vi "Convert to Lockin Data.vi"(8 "error in (no error)":errorcluster, 10 "Raw data":i32[](array[numeric])=[67108864, 0, 0, 67108864, 0, 0, 67108864], 11 "RP Transceiver in":refnum<class "RP Transceiver.lvclass">) -> (0 "error out":errorcluster, 1 "Volatge X out":dbl[](array[numeric]), 2 "Frequency out":dbl[](array[numeric]), 3 "RP Transceiver out":refnum<class "RP Transceiver.lvclass">, 4 "Starting edges":i32[](array[numeric]), 5 "Ending edges":i32[](array[numeric]), 6 "Volatge Y out":dbl[](array[numeric]))   [LabVIEW 2016, in "RP Transceiver.lvclass"]
uses:
  RP Transceiver.lvclass
  RP Transceiver.lvclass/RP Transceiver.ctl
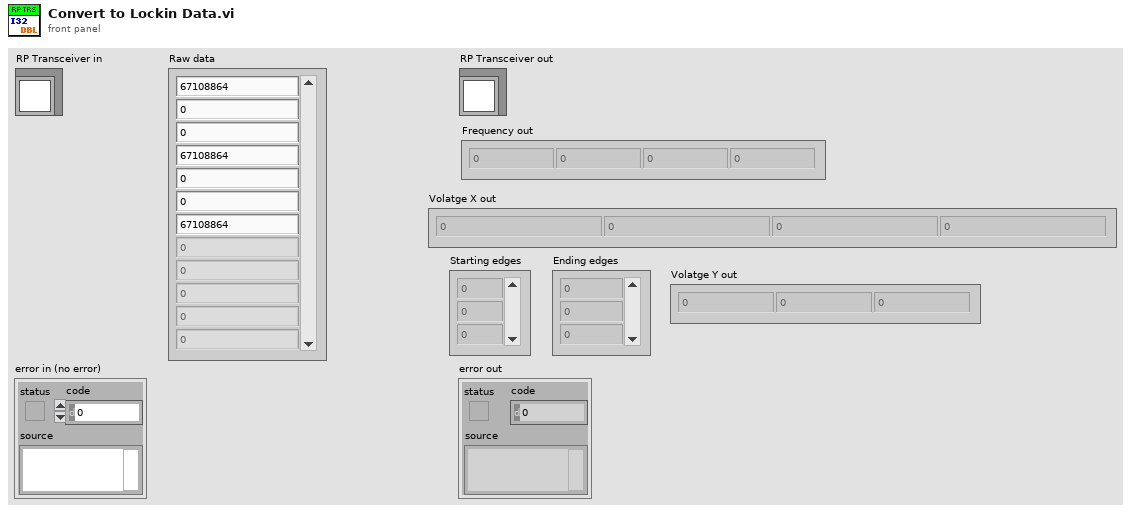
[diagram p1: front panel]
types:
  T1 = typedef "Receiver format.ctl" = enum16{"X-Y-F", "F-X-Y", "X-Y", "X"}
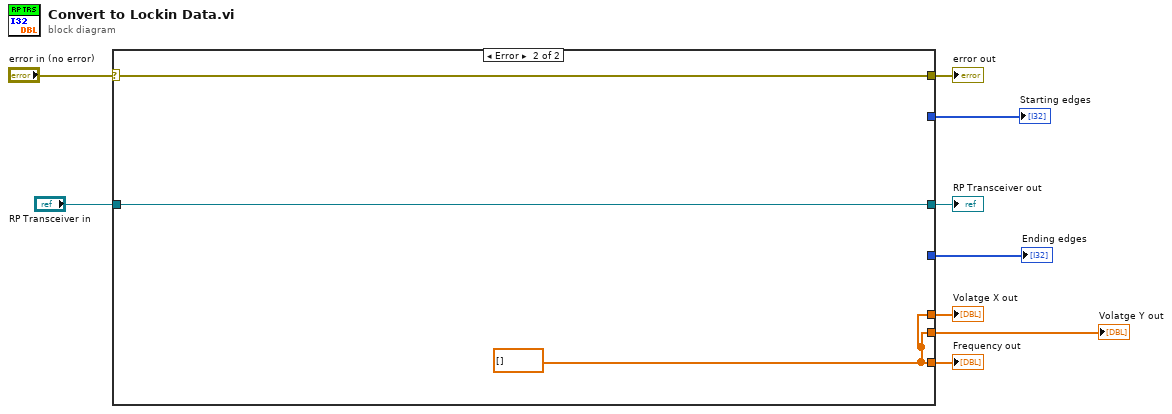
[diagram p0: block diagram]
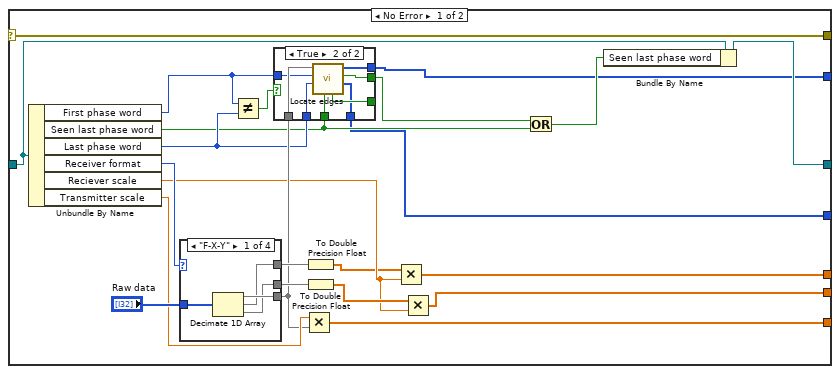
[diagram p2: hidden frame]
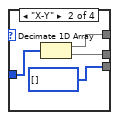
[diagram p4: hidden frame]
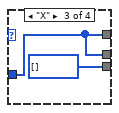
[diagram p5: hidden frame]
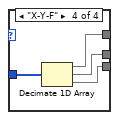
[diagram p6: hidden frame]
diagram:
  n1 = case shown="Error" "error in (no error)" {
    selector: "error in (no error)" -> [w32 w58]
    tunnel: [w32 w58] -> w8
    tunnel: [w23 w57] -> w6
    tunnel: "RP Transceiver in" -> [w27 w57]
    tunnel: [w30 w56] -> w5
    tunnel: [w14 w56] -> w4
    tunnel: [w16 _] -> w3
    tunnel: [w15 _] -> w2
    tunnel: [w10 w56] -> w1
    frame No Error {
      n2 = Unbundle By Name(w27) -> ("First phase word"=w22:i32, "Seen last phase word"=w19:bool, "Last phase word"=w21:i32, "Receiver format"=w25:T1, "Reciever scale"=w12:dbl, "Transmitter scale"=w26:dbl)
      n3 = case shown="\"F-X-Y\"" w25 {
        tunnel: "Raw data" -> [w45 w49 w50 w55]
        tunnel: [w44 i32[] [] i32[] [] w54] -> w24
        tunnel: [w43 w48 w50 w53] -> w29
        tunnel: [w42 w47 w50 w52] -> w28
        frame "F-X-Y" {
          n4 = Decimate 1D Array(w45) -> (w44:i32[], w43:i32[], w42:i32[])
        }
        frame "X-Y" {
          n5 = Decimate 1D Array(w49) -> (w48:i32[], w47:i32[])
        }
        frame "X" {
        }
        frame "X-Y-F" {
          n6 = Decimate 1D Array(w55) -> (w53:i32[], w52:i32[], w54:i32[])
        }
      }
      n7 = Not Equal?(x=w22, y=w21) -> (x != y?=w20:bool)
      n8 = case shown="True" w20 {
        tunnel: w24 -> [_ w41]
        tunnel: w22 -> [_ w40]
        tunnel: w21 -> [_ w39]
        tunnel: w19 -> [w33 w38]
        tunnel: [w33 w37] -> _
        tunnel: [_ w36] -> w16
        tunnel: [w33 w35] -> w17
        tunnel: [_ w34] -> w15
        frame False {
        }
        frame True {
          n9 = call "Locate edges.vi"("Seen last value"=w38, "Last value"=w39, "First value"=w40, "Values"=w41) -> ("Ending edges"=w34:i32[], "Seen last value 2"=w35:bool, "Starting edges"=w36:i32[], "Seen last value out"=w37:bool)  [unwired: 4 in]
        }
      }
      n10 = Multiply(x=w26, y=w24) -> (x*y=w30:dbl[])
      n11 = To Double Precision Float(number=w29) -> (double precision float=w11:dbl[])
      n12 = To Double Precision Float(number=w28) -> (double precision float=w13:dbl[])
      n13 = Multiply(x=w11, y=w12) -> (x*y=w14:dbl[])
      n14 = Multiply(x=w13, y=w12) -> (x*y=w10:dbl[])
      n15 = Or(x=w17, y=w19) -> (x .or. y?=w18:bool)
      n16 = Bundle By Name(cluster=w27, "Seen last phase word"=w18) -> (w23:refnum<class "RP Transceiver.lvclass">)
    }
    frame Error {
      w56 = dbl[] [] ("Data out")
    }
  }
  "error out" <- w8
  "RP Transceiver out" <- w6
  "Frequency out" <- w5
  "Volatge X out" <- w4
  "Ending edges" <- w2
  "Starting edges" <- w3
  "Volatge Y out" <- w1
